vi "Verileri GUI'ye Gönder_Guc.vi"(3 "Uygulanan Değerler":dbl[][](array[numeric])=[[0.0, 0.0, 0.0, 0.0], [0.0, 0.0, 0.0, 0.0]], 4 "FD2 C":dbl, 5 "FD2 B":dbl, 6 "FD2 A":dbl, 7 "FD1 C":dbl, 8 "FD1 B":dbl, 9 "FD1 A":dbl, 10 "Limit Deger":dbl, 11 "Ölçüm No":u16) -> ()   [LabVIEW 2014]
uses:
  VeriPaylasim_Globali.vi
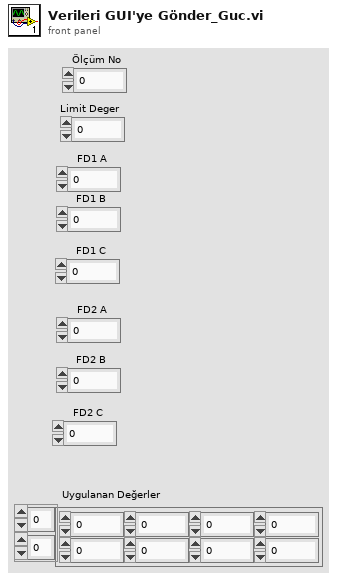
[diagram p1: front panel]
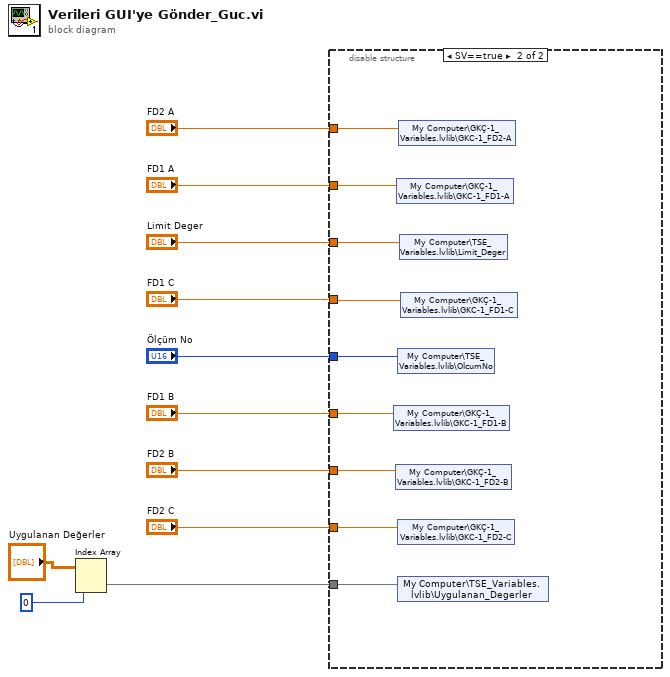
[diagram p0: block diagram]
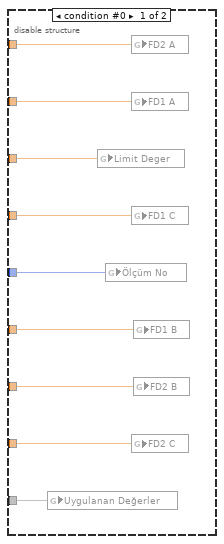
[diagram p2: hidden frame]
diagram:
  n1 = Index Array(array="Uygulanan Değerler", index (row)=0) -> (element=w1:dbl[])  [unwired: 1 in]
  n2 = disable-structure shown="SV==true" {
    disable-tunnel: "FD1 C" -> [w20 w26]
    disable-tunnel: "Limit Deger" -> [w19 w27]
    disable-tunnel: "FD2 A" -> [w18 w29]
    disable-tunnel: "FD1 A" -> [w17 w28]
    disable-tunnel: "Ölçüm No" -> [w16 w25]
    disable-tunnel: "FD1 B" -> [w15 w24]
    disable-tunnel: "FD2 B" -> [w14 w23]
    disable-tunnel: "FD2 C" -> [w13 w22]
    disable-tunnel: w1 -> [w12 w21]
    frame condition #0 {
      n3 = global write "VeriPaylasim_Globali.vi" "Uygulanan Değerler"(w12) -> ()
      n4 = global write "VeriPaylasim_Globali.vi" "Limit Deger"(w19) -> ()
      n5 = global write "VeriPaylasim_Globali.vi" "Ölçüm No"(w16) -> ()
      n6 = global write "VeriPaylasim_Globali.vi" "FD2 A"(w18) -> ()
      n7 = global write "VeriPaylasim_Globali.vi" "FD1 A"(w17) -> ()
      n8 = global write "VeriPaylasim_Globali.vi" "FD1 C"(w20) -> ()
      n9 = global write "VeriPaylasim_Globali.vi" "FD2 C"(w13) -> ()
      n10 = global write "VeriPaylasim_Globali.vi" "FD1 B"(w15) -> ()
      n11 = global write "VeriPaylasim_Globali.vi" "FD2 B"(w14) -> ()
    }
    frame condition #1 (active) {
      n12 = shared-variable "My Computer\\GKÇ-1_Variables.lvlib\\GKC-1_FD1-B"(w24) -> ()  [unwired: 1 in, 1 out]
      n13 = shared-variable "My Computer\\GKÇ-1_Variables.lvlib\\GKC-1_FD2-B"(w23) -> ()  [unwired: 1 in, 1 out]
      n14 = shared-variable "My Computer\\GKÇ-1_Variables.lvlib\\GKC-1_FD1-A"(w28) -> ()  [unwired: 1 in, 1 out]
      n15 = shared-variable "My Computer\\TSE_Variables.lvlib\\OlcumNo"(w25) -> ()  [unwired: 1 in, 1 out]
      n16 = shared-variable "My Computer\\GKÇ-1_Variables.lvlib\\GKC-1_FD2-C"(w22) -> ()  [unwired: 1 in, 1 out]
      n17 = shared-variable "My Computer\\TSE_Variables.lvlib\\Uygulanan_Degerler"(w21) -> ()  [unwired: 1 in, 1 out]
      n18 = shared-variable "My Computer\\GKÇ-1_Variables.lvlib\\GKC-1_FD2-A"(w29) -> ()  [unwired: 1 in, 1 out]
      n19 = shared-variable "My Computer\\TSE_Variables.lvlib\\Limit_Deger"(w27) -> ()  [unwired: 1 in, 1 out]
      n20 = shared-variable "My Computer\\GKÇ-1_Variables.lvlib\\GKC-1_FD1-C"(w26) -> ()  [unwired: 1 in, 1 out]
    }
  }
